vi "insert.vi"(8 "error in (no error)":errorcluster, 11 "DL090211FrameImageAssembler in":refnum<class "ImageAssemblerDL090211Frame.lvclass">) -> (0 "error out":errorcluster, 3 "DL090211FrameImageAssembler out":refnum<class "ImageAssemblerDL090211Frame.lvclass">)   [LabVIEW 2010, in "ImageAssemblerDL090211Frame.lvclass"]
uses:
  ImageAssemblerDL090211Frame.lvclass
  ImageAssemblerDL090211Frame.lvclass/ImageAssemblerDL090211Frame.ctl
  common/classes/Image/Image/Image.lvclass
  ImageAssemblerDL090211Scaffold/ImageAssemblerDL090211Scaffold/ImageAssemblerDL090211Scaffold.lvclass
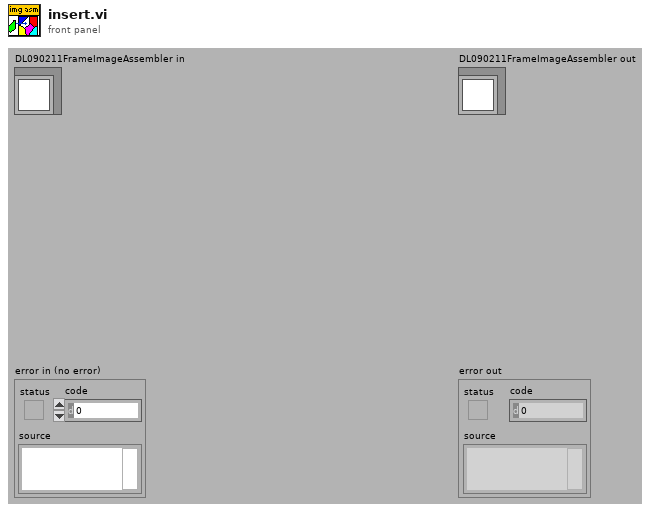
[diagram p1: front panel]
types:
  T1 = typedef "pixel_raw_data_array.ctl" = dbl[][]
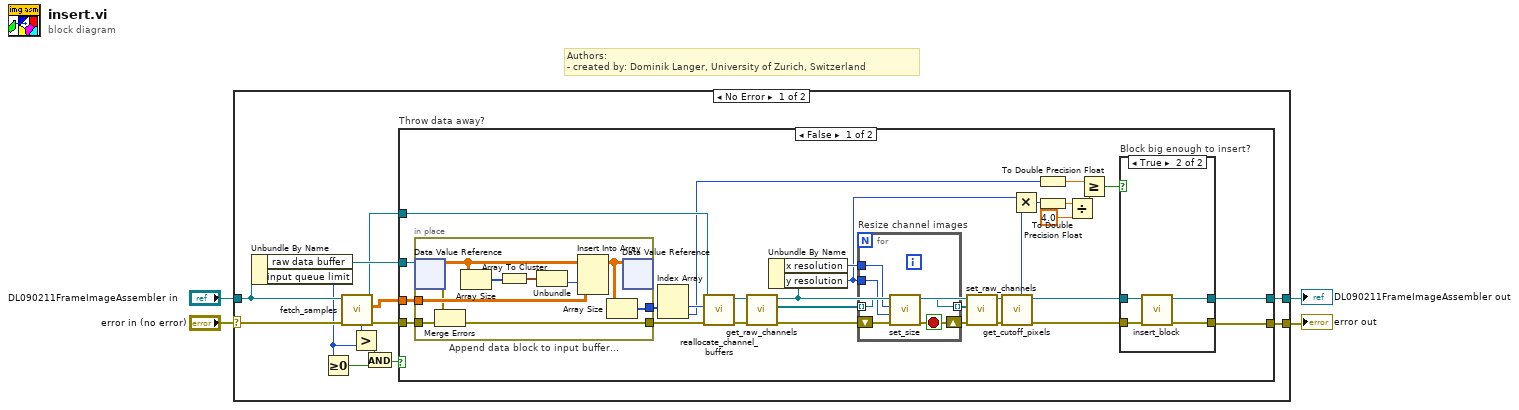
[diagram p0: block diagram]
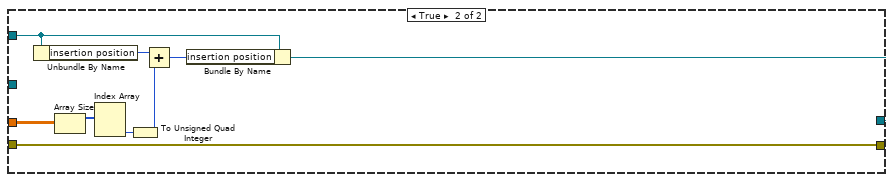
[diagram p3: hidden frame]
diagram:
  # "Authors: \n- created by: Dominik Langer, University of Zurich, Switzerland"
  n1 = case shown="No Error" "error in (no error)" {
    selector: "error in (no error)" -> [w14 w79]
    tunnel: "DL090211FrameImageAssembler in" -> [w13 w80]
    tunnel: [w17 w79] -> w4
    tunnel: [w16 w80] -> w3
    frame No Error {
      n2 = Unbundle By Name(w13) -> ("raw data buffer"=w15:refnum<data-value>, "input queue limit"=w11:i32)
      n3 = Greater Or Equal To 0?(x=w11) -> (x >= 0?=w10:bool)
      n4 = call-dynamic "fetch_samples.vi"("error in (no error)"=w14, "GenericToplevelComponent in"=w13) -> ("error out"=w6:errorcluster, "channels raw data block"=w5:T1, "GenericToplevelComponent out"=w12:refnum<class "ImageAssemblerDL090211Frame.lvclass">, "# elements in queue"=w9:i32)  [unwired: 6 in]
      n5 = Greater?(x=w9, y=w11) -> (0:w8:bool)
      n6 = And(x=w8, y=w10) -> (x .and. y?=w7:bool)
      n7 = case "Throw data away?" shown="False" w7 {
        tunnel: [w47 w74] -> w17
        tunnel: [w46 w73] -> w16
        tunnel: w15 -> [w45 _]
        tunnel: w12 -> [w43 w71]
        tunnel: w5 -> [w30 w75]
        tunnel: w6 -> [w29 w74]
        frame False {
          n8 = in-place "Append data block to input buffer..." {
            in-place-border: w30 -> [w55]
            in-place-border: w29 -> [w52]
            in-place-border: [w50] -> w44
            in-place-border: [w48] -> w28
            n9 = in-place-dvr #1(w45) -> (w53:T1, w51:errorcluster)
            n10 = Merge Errors(w51, w52) -> (w50:errorcluster)
            n11 = Array Size(array=w53) -> (size(s)=w57:i32[])
            n12 = Array To Cluster(array=w57) -> (cluster=w56:cluster{"[0]":i32, "[1]":i32})
            n13 = Unbundle(w56) -> ("[1]"=w54:i32)  [unwired: 1 out]
            n14 = Insert Into Array(array=w53, index (col)=w54, new element=w55) -> (w49:T1)  [unwired: 1 in]
            n15 = Array Size(array=w49) -> (size(s)=w48:i32[])
            n16 = in-place-dvr #1(w49) -> ()  [unwired: 2 out]
          }
          n17 = Index Array(array=w28) -> (element #1=w42:i32, element #2=w21:i32)  [unwired: 2 in]
          n18 = call-dynamic "reallocate_channel_buffers.vi"("error in (no error)"=w44, "new size"=w42, "ImageAssemblerDL090211Scaffold in"=w43) -> ("error out"=w36:errorcluster, "ImageAssemblerDL090211Scaffold out"=w35:refnum<class "ImageAssemblerDL090211Frame.lvclass">)  [unwired: 7 in]
          n19 = call-dynamic "get_raw_channels.vi"("error in (no error)"=w36, "DL090211ImageAssemblerScaffold.lvclass in"=w35) -> ("error out"=w38:errorcluster, "raw channels"=w39:refnum<class "Image.lvclass">[], "DL090211ImageAssemblerScaffold.lvclass out"=w37:refnum<class "ImageAssemblerDL090211Frame.lvclass">)  [unwired: 7 out]
          n20 = Unbundle By Name(w37) -> ("x resolution"=w23:i32, "y resolution"=w18:i32)
          n21 = for "Resize channel images" {
            shift-right: [w58] -> w40
            shift-left: w38 -> [w63]
            tunnel: w39 -> [w62] mode=indexing
            tunnel: w23 -> [w60]
            tunnel: w18 -> [w61]
            tunnel: [w59] -> w41 mode=indexing
            stop <- w58 stop-if-true
            n22 = call-dynamic "set_size.vi"("error in (no error)"=w63, "y"=w61, "x"=w60, "Image in"=w62) -> ("error out"=w58:errorcluster, "Image out"=w59:refnum<class "Image.lvclass">)  [unwired: 6 out]
          }
          n23 = call "set_raw_channels.vi"("error in (no error)"=w40, "raw channels"=w41, "DL090211ImageAssemblerScaffold.lvclass in"=w37) -> ("error out"=w34:errorcluster, "DL090211ImageAssemblerScaffold.lvclass out"=w31:refnum<class "ImageAssemblerDL090211Frame.lvclass">)  [unwired: 7 out]
          n24 = call-dynamic "get_cutoff_pixels.vi"("error in (no error)"=w34, "DL090211FrameImageAssembler in"=w31) -> ("error out"=w33:errorcluster, "DL090211FrameImageAssembler out"=w32:refnum<class "ImageAssemblerDL090211Frame.lvclass">, "total pixels per line"=w27:i32)  [unwired: 7 out]
          n25 = Multiply(x=w18, y=w27) -> (x*y=w26:i32)
          n26 = To Double Precision Float(number=w21) -> (double precision float=w20:dbl)
          n27 = To Double Precision Float(number=w26) -> (double precision float=w25:dbl)
          n28 = Divide(x=w25, y=4.0) -> (x/y=w22:dbl)
          n29 = Greater Or Equal?(x=w20, y=w22) -> (x >= y?=w19:bool)
          n30 = case "Block big enough to insert?" shown="True" w19 {
            tunnel: [w64 w66] -> w47
            tunnel: [w65 w67] -> w46
            tunnel: w33 -> [w64 w69]
            tunnel: w32 -> [w65 w68]
            frame False {
            }
            frame True {
              n31 = call-dynamic "insert_block.vi"("error in (no error)"=w69, "ImageAssemblerDL090211Frame in"=w68) -> ("error out"=w66:errorcluster, "ImageAssemblerDL090211Frame out"=w67:refnum<class "ImageAssemblerDL090211Frame.lvclass">)  [unwired: 8 in]
            }
          }
        }
        frame True {
          n32 = Unbundle By Name(w71) -> ("insertion position"=w70:u64)
          n33 = Array Size(array=w75) -> (size(s)=w78:i32[])
          n34 = Index Array(array=w78) -> (element #2=w77:i32)  [unwired: 2 in, 1 out]
          n35 = To Unsigned Quad Integer(1:w77) -> (0:w76:u64)
          n36 = Add(x=w70, y=w76) -> (x+y=w72:u64)
          n37 = Bundle By Name(cluster=w71, "insertion position"=w72) -> (w73:refnum<class "ImageAssemblerDL090211Frame.lvclass">)
        }
      }
    }
    frame Error {
    }
  }
  "error out" <- w4
  "DL090211FrameImageAssembler out" <- w3
